vi "Lock-in measure R with auto sensitivity.vi"(8 "error in (no error)":errorcluster, 10 "seconds to wait":u32, 11 "Instrument parameters":T1) -> (0 "error out":errorcluster, 2 "Data out":dbl, 3 "output cluster":T1)   [LabVIEW 2016, in "MyLockIn.lvlib"]
uses:
  MyLockIn.lvlib
  TYPE DEFS/S2DS_Instrument parameters.ctl
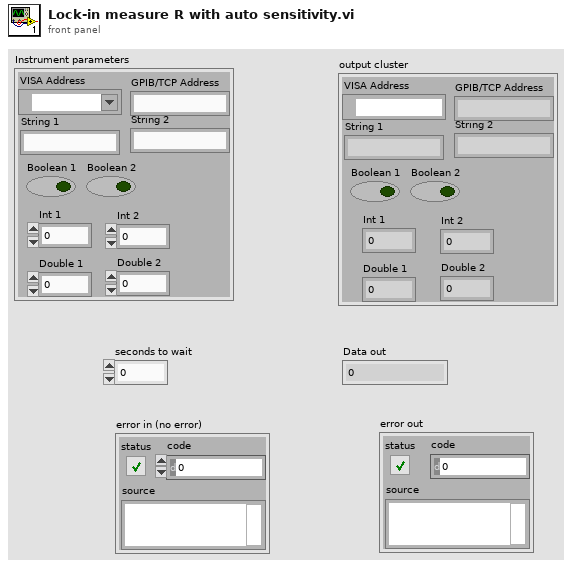
[diagram p1: front panel]
types:
  T1 = typedef "S2DS_Instrument parameters.ctl" = cluster{"VISA Address":refnum<visa-resource-name>, "GPIB/TCP Address":string, "String 1":string, "String 2":string, "Boolean 1":bool, "Boolean 2":bool, "Int 1":i32, "Int 2":i32, "Double 1":dbl, "Double 2":dbl}
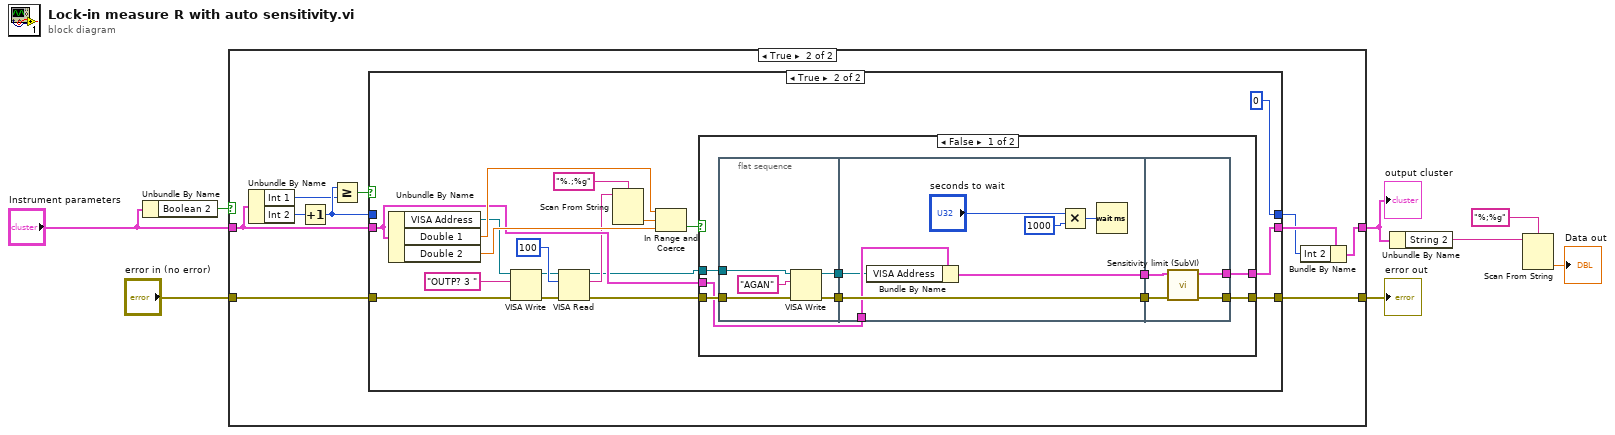
[diagram p0: block diagram]
diagram:
  n1 = Unbundle By Name("Instrument parameters") -> ("Boolean 2"=w7:bool)
  n2 = case shown="True" w7 {
    tunnel: [w9 w20] -> w8
    tunnel: "Instrument parameters" -> [w10 w17]
    tunnel: [w10 w12] -> w4
    tunnel: "error in (no error)" -> [w9 w11]
    frame False {
    }
    frame True {
      n3 = Unbundle By Name(w17) -> ("Int 1"=w16:i32, "Int 2"=w15:i32)
      n4 = Increment(x=w15) -> (x+1=w18:i32)
      n5 = Greater Or Equal?(x=w18, y=w16) -> (x >= y?=w19:bool)
      n6 = case shown="True" w19 {
        tunnel: [w22 w40] -> w20
        tunnel: w11 -> [w22 w28]
        tunnel: [w23 0] -> w13
        tunnel: w18 -> [w23 _]
        tunnel: w17 -> [w21 w36]
        tunnel: [w21 w35] -> w14
        frame False {
        }
        frame True {
          n7 = Unbundle By Name(w36) -> ("VISA Address"=w24:refnum<visa-resource-name>, "Double 1"=w38:dbl, "Double 2"=w37:dbl)
          n8 = VISA Write(VISA resource name=w24, write buffer="OUTP? 3 " ("initial string"), error in (no error)=w28) -> (VISA resource name out=w31:refnum<visa-resource-name>, error out=w30:errorcluster)  [unwired: 1 out]
          n9 = VISA Read(VISA resource name=w31, byte count=u32 100, error in (no error)=w30) -> (VISA resource name out=w26:refnum<visa-resource-name>, read buffer=w29:string, error out=w27:errorcluster)  [unwired: 1 out]
          n10 = Scan From String(format string="%.;%g", input string=w29) -> (output 1=w25:dbl)  [unwired: 3 in, 3 out]
          n11 = In Range and Coerce(upper limit=w38, x=w25, lower limit=w37) -> (In Range?=w41:bool)  [unwired: 1 out]
          n12 = case shown="False" w41 {
            tunnel: w26 -> [w50 _]
            tunnel: w27 -> [w48 w68]
            tunnel: [w45 w68] -> w40
            tunnel: w36 -> [w43 w67]
            tunnel: [w42 w67] -> w35
            frame False {
              n13 = flat-sequence {
                tunnel: w50 -> [w54]
                tunnel: [w53] -> w49
                tunnel: w48 -> [w52]
                tunnel: [w51] -> w46
                tunnel: w49 -> [w56]
                tunnel: [w59] -> w47
                tunnel: w46 -> [w59]
                tunnel: [w57] -> w44
                tunnel: w43 -> [w58]
                tunnel: [w66] -> w45
                tunnel: [w63] -> w42
                tunnel: w44 -> [w64]
                tunnel: w47 -> [w65]
                frame #0 {
                  n14 = VISA Write(VISA resource name=w54, write buffer="AGAN", error in (no error)=w52) -> (VISA resource name out=w53:refnum<visa-resource-name>, error out=w51:errorcluster)  [unwired: 1 out]
                }
                frame #1 {
                  n15 = Bundle By Name(cluster=w58, "VISA Address"=w56) -> (w57:T1)
                  n16 = Multiply(x="seconds to wait", y=u32 1000) -> (x*y=w60:u32)
                  n17 = Wait (ms)(milliseconds to wait=w60) -> ()  [unwired: 1 out]
                }
                frame #2 {
                  n18 = call "Sensitivity limit (SubVI).vi"("error in (no error)"=w65, "Instrument parameters in"=w64) -> ("error out"=w66:errorcluster, "Instrument parameters out"=w63:T1)  [unwired: 7 in, 1 out]
                }
              }
            }
            frame True {
            }
          }
        }
      }
      n19 = Bundle By Name(cluster=w14, "Int 2"=w13) -> (w12:T1)
    }
  }
  "error out" <- w8
  "output cluster" <- w4
  n20 = Unbundle By Name(w4) -> ("String 2"=w3:string)
  n21 = Scan From String(format string="%;%g", input string=w3) -> (output 1=→"Data out":dbl)  [unwired: 3 in, 3 out]
